vi "Start Process.vi"(0 "Process In":refnum<class "Process.lvclass">, 7 "ms Timeout (-1)":i32=-1, 11 "Error In":errorcluster) -> (4 "Process Out":refnum<class "Process.lvclass">, 8 "Timed Out":bool, 15 "Error In":errorcluster)   [LabVIEW 2023, in "Process.lvclass"]
doc: "Looks up an existing object matching object name or creates a new object and returns a refnum you can use when calling other class methods.\n\nObjects created with this VI should be destroyed using this class Delete VI."
uses:
  Process.lvclass
  Process.lvclass/Process.ctl
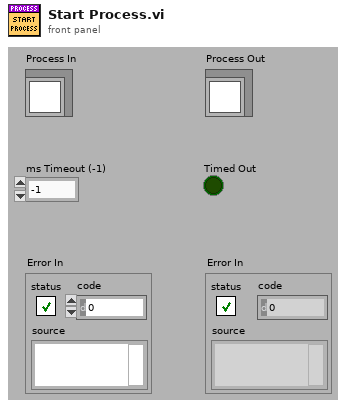
[diagram p1: front panel]
types:
  T1 = enum16{"ReadRepository", "CreateNew", "CreateOrLookUpExisting", "ReadRepositoryAndDestroy"}
  T2 = typedef "ICanCommunicate.lvclass/ProcessSyncQueue.ctl" = refnum<queue>
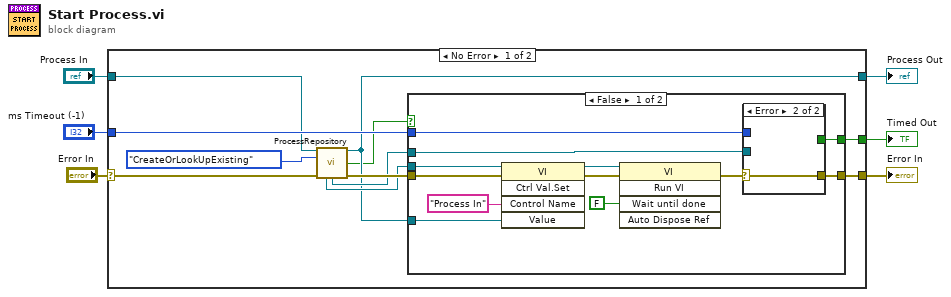
[diagram p0: block diagram]
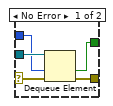
[diagram p2: hidden frame]
diagram:
  n1 = case shown="No Error" "Error In" {
    selector: "Error In" -> [w14 w37]
    tunnel: [w15 w37] -> w5
    tunnel: [w10 w38] -> w3
    tunnel: "Process In" -> [w8 w38]
    tunnel: "ms Timeout (-1)" -> [w17 _]
    tunnel: [w16 _] -> w1
    frame No Error {
      n2 = call-dynamic "ProcessRepository.vi"("Process In"=w8, "Action(ReadRepository)"=T1."CreateOrLookUpExisting", "Error In"=w14) -> ("Process Out"=w10:refnum<class "Process.lvclass">, "ProcessAlreadyStarted"=w9:bool, "ProcessViRef"=w12:refnum<vi>, "ProcessSyncQueue"=w11:T2, "Error Out"=w13:errorcluster)  [unwired: 6 in, 2 out]
      n3 = case shown="False" w9 {
        tunnel: w17 -> [w25 _]
        tunnel: [w24 _] -> w16
        tunnel: [w22 w36] -> w15
        tunnel: w13 -> [w21 w36]
        tunnel: w12 -> [w20 _]
        tunnel: w11 -> [w19 _]
        tunnel: w10 -> [w18 _]
        frame False {
          n4 = invoke class="VI" method="Ctrl Val.Set"(reference=w20, error in=w21, "Control Name"="Process In", "Value"=w18) -> (reference out=w28:refnum<vi>, error out=w27:errorcluster)  [unwired: 1 in, 3 out]
          n5 = invoke class="VI" method="Run VI"(reference=w28, error in=w27, "Wait until done"=FALSE ("Wait Until Done")) -> (error out=w23:errorcluster)  [unwired: 2 in, 4 out]
          n6 = case shown="Error" w23 {
            tunnel: w19 -> [w34 _]
            tunnel: w25 -> [w33 _]
            tunnel: [w32 _] -> w24
            selector: w23 -> [w31 w35]
            tunnel: [w30 w35] -> w22
            frame No Error {
              n7 = Dequeue Element(queue=w34, timeout in ms (-1)=w33, error in (no error)=w31) -> (timed out?=w32:bool, error out=w30:errorcluster)  [unwired: 2 out]
            }
            frame Error {
            }
          }
        }
        frame True {
          # "Process Already started.\nThis option will only be used togeather with the\naction: \"CreateOrLookUpExisting\""
        }
      }
    }
    frame Error {
    }
  }
  "Error In" <- w5
  "Process Out" <- w3
  "Timed Out" <- w1
